vi "Save.vi"(8 "error in (no error)":errorcluster, 9 "new command":string, 10 "Msg in":T1, 11 "FakePressureController in":refnum<class "Ztec4611.lvclass">) -> (0 "error out":errorcluster, 1 "Path":path, 2 "Msg out":T1, 3 "FakePressureController out":refnum<class "Ztec4611.lvclass">, 4 "new command":string)   [LabVIEW 2011, in "Ztec4611.lvclass"]
uses:
  Ztec4611.lvclass
  DriverMsg.ctl
  Ztec4611.lvclass/Ztec4611.ctl
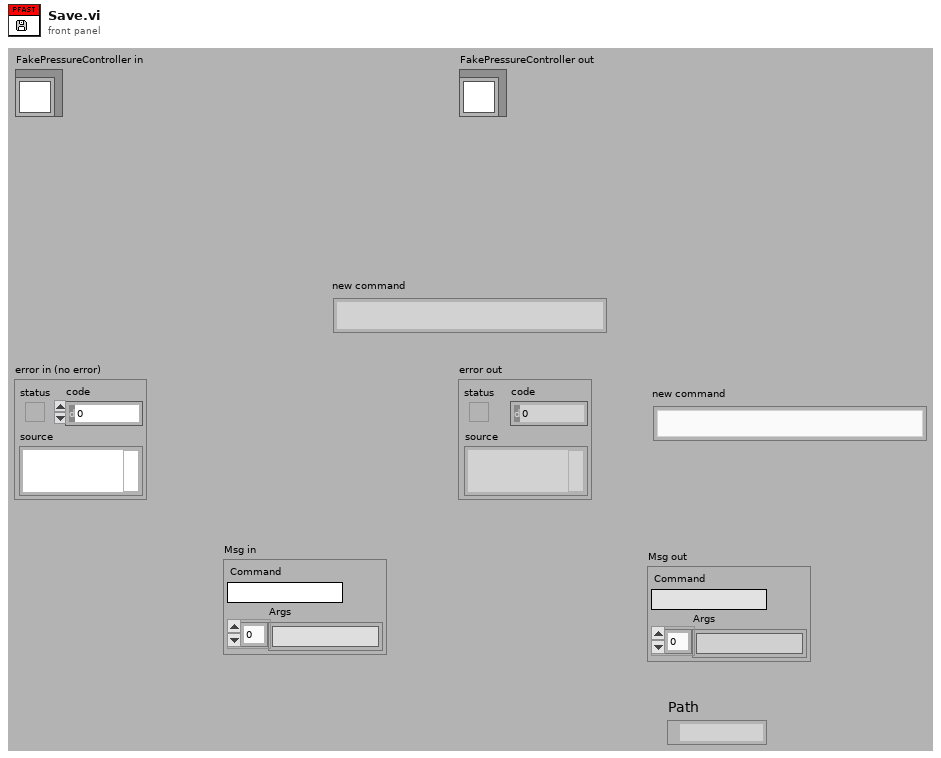
[diagram p1: front panel]
types:
  T1 = typedef "DriverMsg.ctl" = cluster{"Command":string, "Args":string[]}
  T2 = cluster{"actualSamples":i32, "absoluteInitialX":dbl, "relativeInitialX":dbl, "xIncrement":dbl, "offset":dbl, "gain":dbl, "reserved1":dbl, "reserved2":dbl}[]
  T3 = typedef "ScopeTrace_String_TypDef.ctl" = cluster{"Channel0":string, "Channel1":string, "Channel2":string, "Channel3":string, "Channel5":string, "Channel4":string, "Channel6":string, "Channel7":string}
  T4 = typedef "channelenabled_TypDef.ctl" = cluster{"Channel0":T5, "Channel1":T5, "Channel2":T5, "Channel3":T5, "Channel4":T5, "Channel5":T5, "Channel6":T5, "Channel7":T5}
  T5 = typedef "OnOffTypeDef.ctl" = enum16{"off", "on"}
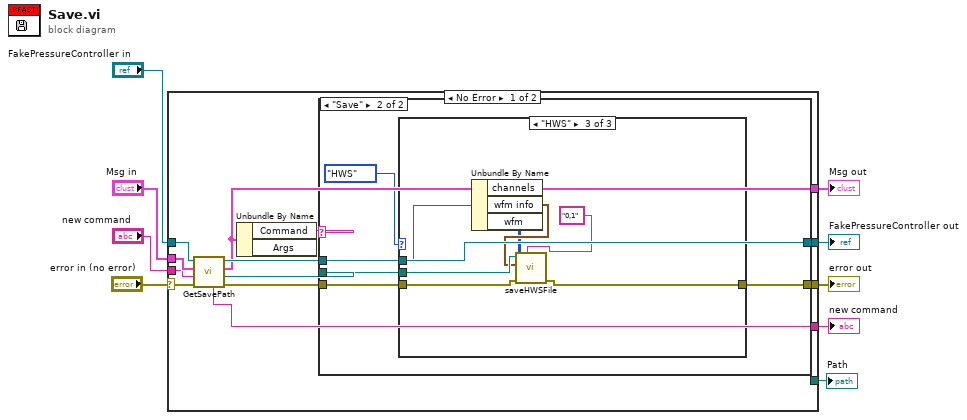
[diagram p0: block diagram]
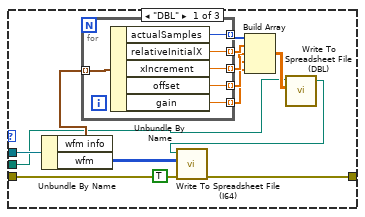
[diagram p3: hidden frame]
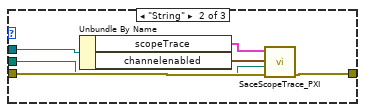
[diagram p4: hidden frame]
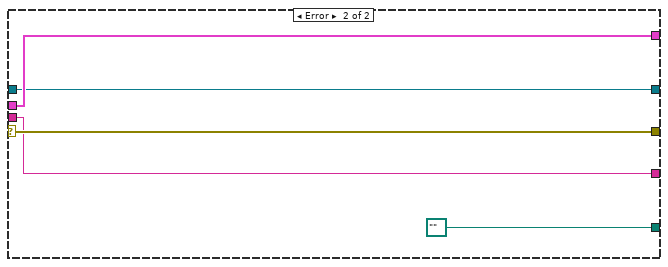
[diagram p5: hidden frame]
diagram:
  n1 = case shown="No Error" "error in (no error)" {
    selector: "error in (no error)" -> [w15 w65]
    tunnel: [w19 w65] -> w5
    tunnel: [_ path "" ("Path")] -> w1
    tunnel: [w13 w64] -> w6
    tunnel: [w20 w63] -> w8
    tunnel: "Msg in" -> [w17 w64]
    tunnel: "FakePressureController in" -> [w18 w63]
    tunnel: "new command" -> [w16 w61]
    tunnel: [w10 w61] -> w2
    frame No Error {
      n2 = call-dynamic "GetSavePath.vi"("error in (no error)"=w15, "new command"=w16, "Msg in"=w17, "BaseDriver in"=w18) -> ("error out"=w11:errorcluster, "Path"=w12:path, "Msg out"=w13:T1, "BaseDriver out"=w14:refnum<class "Ztec4611.lvclass">, "new command"=w10:string)  [unwired: 3 in]
      n3 = Unbundle By Name(w13) -> ("Command"=w21:string)  [unwired: 1 out]
      n4 = case shown="\"Save\"" w21 {
        tunnel: w14 -> [w23 w28]
        tunnel: [w23 w28] -> w20
        tunnel: w12 -> [_ w25]
        tunnel: w11 -> [w22 w27]
        tunnel: [w22 w26] -> w19
        frame Default {
        }
        frame "Save" {
          n5 = case shown="\"HWS\"" enum16{"String", "DBL", "HWS"}."HWS" ("Sving Method") {
            tunnel: w28 -> [w41 w53 w60]
            tunnel: w27 -> [w40 w52 w56]
            tunnel: [w40 w51 w55] -> w26
            tunnel: w25 -> [w31 w49 w59]
            frame "DBL" {
              n6 = Unbundle By Name(w41) -> ("wfm info"=w38:T2, "wfm"=w39:i16[][])
              n7 = for {
                tunnel: w38 -> [w47] mode=indexing
                tunnel: [w46] -> w37 mode=indexing
                tunnel: [w45] -> w36 mode=indexing
                tunnel: [w44] -> w35 mode=indexing
                tunnel: [w43] -> w34 mode=indexing
                tunnel: [w42] -> w33 mode=indexing
                n8 = Unbundle By Name(w47) -> ("actualSamples"=w46:i32, "relativeInitialX"=w45:dbl, "xIncrement"=w44:dbl, "offset"=w43:dbl, "gain"=w42:dbl)
              }
              n9 = Build Array(w37, w36, w35, w34, w33) -> (w32:dbl[][])
              n10 = call "Write To Spreadsheet File (DBL).vi"("2D data"=w32, "file path (dialog if empty)"=w31) -> ("new file path (Not A Path if cancelled)"=w30:path)  [unwired: 6 in]
              n11 = call "Write To Spreadsheet File (I64).vi"("append to file? (new file:F)"=TRUE, "2D data"=w39, "file path (dialog if empty)"=w30) -> ()  [unwired: 5 in, 1 out]
            }
            frame "String" {
              n12 = Unbundle By Name(w53) -> ("scopeTrace"=w50:T3, "channelenabled"=w48:T4)
              n13 = call "SaceScopeTrace_PXI.vi"("error in (no error)"=w52, "Path"=w49, "Settings.channelenabled"=w48, "scopeTrace"=w50) -> ("error out"=w51:errorcluster)  [unwired: 7 in]
            }
            frame "HWS" {
              n14 = Unbundle By Name(w60) -> ("wfm info"=w58:T2, "wfm"=w57:i16[][])  [unwired: 1 out]
              n15 = call "saveHWSFile.vi"("active channels (aqu)"="0,1", "error in (no error)"=w56, "wfm"=w57, "wfm info"=w58, "Destination HWS File"=w59) -> ("error out"=w55:errorcluster)  [unwired: 6 in]
            }
          }
        }
      }
    }
    frame Error {
    }
  }
  "error out" <- w5
  "FakePressureController out" <- w8
  "Path" <- w1
  "Msg out" <- w6
  "new command" <- w2
